vi "Update Global Vars.vi"(8 "Error In":errorcluster, 11 "Cluster in":refnum<vi>) -> (0 "Error Out":errorcluster)   [LabVIEW 2014]
uses:
  Scan Parameters Global Variable.vi
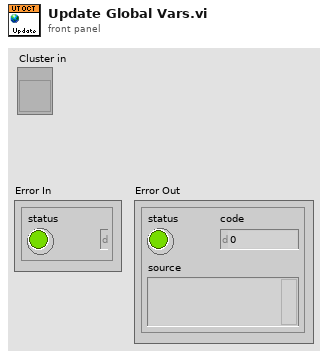
[diagram p1: front panel]
types:
  T1 = typedef "Galvo.lvclass/Scanning Cluster.ctl" = cluster{"Fast Axis Offset":sgl, "Slow Axis Offset":sgl, "Slow Axis Amp":sgl, "Fast Axis Amp":sgl, "Scan Pattern":enum16{"Raster"}}
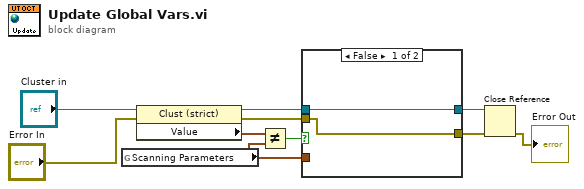
[diagram p0: block diagram]
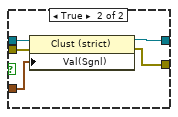
[diagram p2: hidden frame]
diagram:
  n1 = global read "Scan Parameters Global Variable.vi" "Scanning Parameters"() -> (w9:T1)
  n2 = property class="Clust (strict)"(reference="Cluster in", error in="Error In") -> (reference out=w8:refnum<vi>, error out=w4:errorcluster, "Value"=w6:T1)
  n3 = Not Equal?(x=w6, y=w9) -> (x != y?=w7:bool)
  n4 = case shown="False" w7 {
    tunnel: w8 -> [w12 w17]
    tunnel: w9 -> [_ w16]
    tunnel: [w12 w15] -> w10
    tunnel: w4 -> [w11 w14]
    tunnel: [w11 w13] -> w2
    frame False {
    }
    frame True {
      n5 = property class="Clust (strict)"(reference=w17, error in=w14, "Val(Sgnl)"=w16) -> (reference out=w15:refnum<vi>, error out=w13:errorcluster)
    }
  }
  n6 = Close Reference(reference=w10, error in (no error)=w2) -> (error out=→"Error Out":errorcluster)
